vi "Global_Vision Status.vi"() -> ()   [LabVIEW 2017, in "VisionSystem.lvlib"]
uses:
  VisionSystem.lvlib
  Cluster_Vision Status.ctl
  Enum_ Field Targets.ctl
  <vilib>/vision/Image Controls.llb/IMAQ Image.ctl
panel:
  in  "Vison_Final Image":T1
  in  "Vision Status":T2
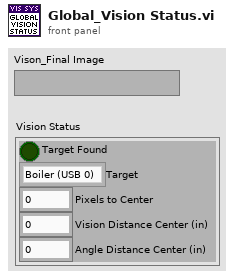
[diagram p1: front panel]
types:
  T1 = typedef "IMAQ Image.ctl" = refnum<image>
  T2 = typedef "VisionSystem.lvlib/Cluster_Vision Status.ctl" = cluster{"Target Found":bool, "Target":T3, "Pixels to Center":dbl, "Vision Distance Center (in)":dbl, "Angle Distance Center (in)":dbl}
  T3 = typedef "VisionSystem.lvlib/Enum_ Field Targets.ctl" = enum16{"Boiler (USB 0)", "Rope (USB 1)"}
diagram:
